vi "Verify Fiducial Positions.vi"(8 "error in":errorcluster, 10 "Module Fiducials":T5(array[cluster])) -> (0 "error out":errorcluster, 2 "All Good":bool)   [LabVIEW 2011]
uses:
  Shared Components/Utils/Type Definitions/Fiducial Image.ctl
  Shared Components/Vec3d Class/Vec3d Class.lvclass
  Shared Components/Utils/Type Definitions/Physical Image.ctl
  <vilib>/vision/Image Controls.llb/IMAQ Image.ctl
  Shared Components/Utils/Type Definitions/Fiducial with Source.ctl
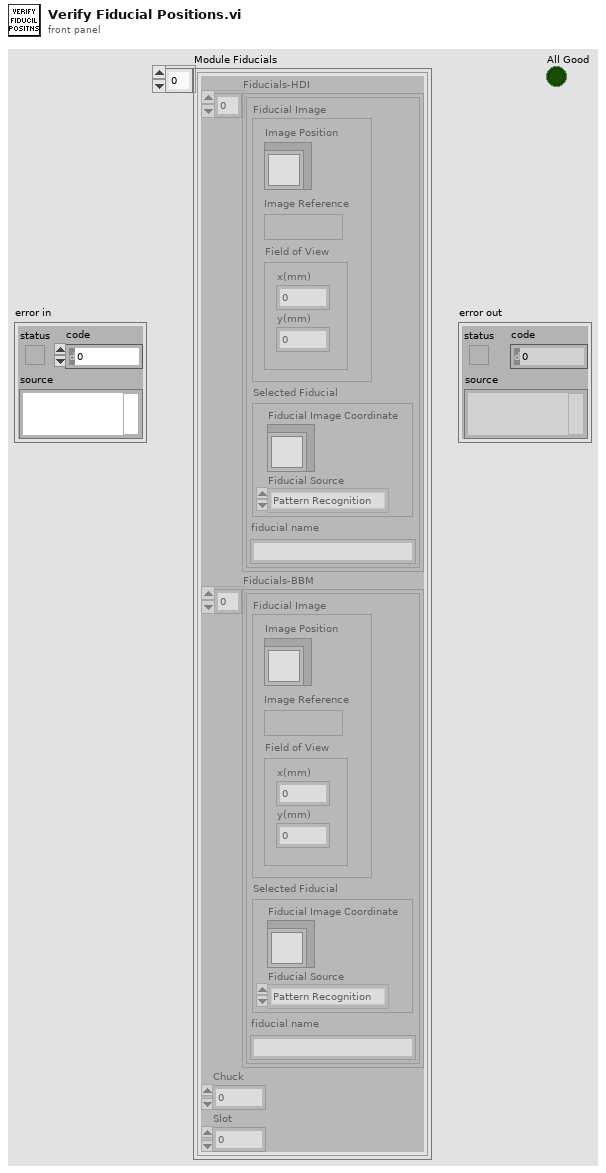
[diagram p1: front panel]
types:
  T1 = typedef "Fiducial Image.ctl" = cluster{"Fiducial Image":T2, "Selected Fiducial":T4, "fiducial name":string}
  T2 = typedef "Physical Image.ctl" = cluster{"Image Position":refnum<class "Vec3d Class.lvclass">, "Image Reference":T3, "Field of View":cluster{"x(mm)":dbl, "y(mm)":dbl}}
  T3 = typedef "IMAQ Image.ctl" = refnum<image>
  T4 = typedef "Fiducial with Source.ctl" = cluster{"Fiducial Image Coordinate":refnum<class "Vec3d Class.lvclass">, "Fiducial Source":enum16{"Pattern Recognition", "User", "Error", "Default"}}
  T5 = cluster{"Fiducials-HDI":T1[], "Fiducials-BBM":T1[], "Chuck":i32, "Slot":i32}[]
  T6 = enum16{"Pattern Recognition", "User", "Error", "Default"}
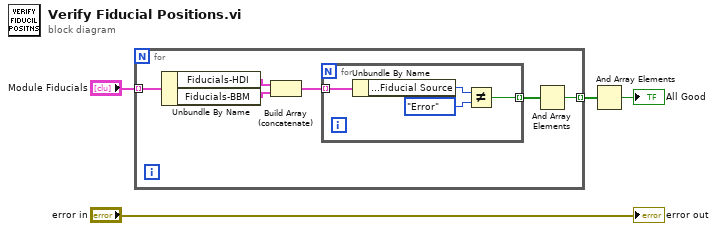
[diagram p0: block diagram]
diagram:
  n1 = for {
    tunnel: "Module Fiducials" -> [w10] mode=indexing
    tunnel: [w5] -> w3 mode=indexing
    n2 = Unbundle By Name(w10) -> ("Fiducials-HDI"=w9:T1[], "Fiducials-BBM"=w8:T1[])
    n3 = Build Array (concatenate)(w9, w8) -> (w7:T1[])
    n4 = for {
      tunnel: w7 -> [w14] mode=indexing
      tunnel: [w12] -> w6 mode=indexing
      n5 = Unbundle By Name(w14) -> ("Selected Fiducial.Fiducial Source"=w13:T6)
      n6 = Not Equal?(x=w13, y=T6."Error") -> (x != y?=w12:bool)
    }
    n7 = And Array Elements(Boolean array=w6) -> (logical AND=w5:bool)
  }
  n8 = And Array Elements(Boolean array=w3) -> (logical AND=→"All Good":bool)
  "error out" <- "error in"
